vi "数组大小.vi"() -> ()   [LabVIEW 2018]
panel:
  in  "停止":bool
  out "大小":i32[](array[numeric])
  in  "数组":dbl[][](array[numeric])
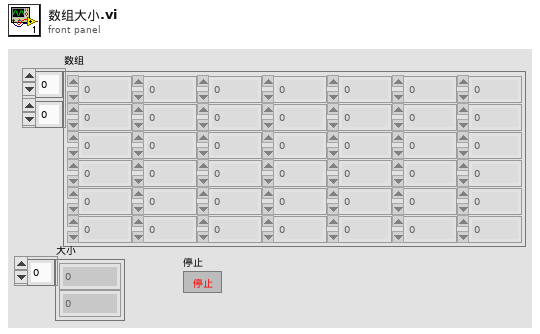
[diagram p1: front panel]
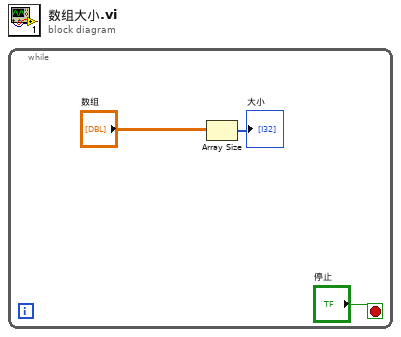
[diagram p0: block diagram]
diagram:
  n1 = while {
    stop <- "停止" stop-if-true
    n2 = Array Size(array="数组") -> (size(s)=→"大小":i32[])
  }
